vi "Periodic Tasks.vi"(8 "error in":errorcluster) -> ()   [LabVIEW 2015]
doc: "This VI runs in parallel to other tasks. It can contain as many user-defined periodic loops as you need. These can carry out PID or other sorts of timed response."
uses:
  <vilib>/Rock Robotics/WPI/Solenoid/Deprecated/WPI_SolenoidSetBool.vi
  <vilib>/Rock Robotics/WPI/Solenoid/Deprecated/WPI_SolenoidGetBool.vi
panel:
  in  "Left Art":dbl=0.5 format="%#_13g"
  in  "Right Art":dbl=0.5 format="%#_13g"
  in  "velocity_lower":dbl=1.0 format="%#_13g"
  in  "velocity_upper":dbl=1.0 format="%#_13g"
  out "error out":errorcluster
  # "change in time in milliseconds"
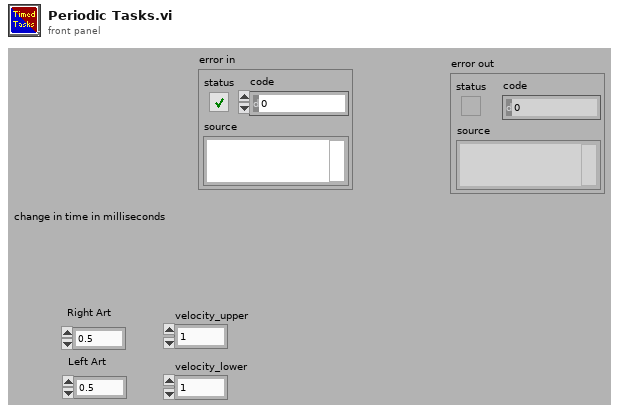
[diagram p1: front panel]
types:
  T1 = typedef "WPI_DigitalInputDevRef.ctl" = cluster{"DevStatus":errorcluster, "DIO Channel":T2}
  T2 = typedef "FPGA_DIOChannel.ctl" = enum8{"DIO 0", "DIO 1", "DIO 2", "DIO 3", "DIO 4", "DIO 5", "DIO 6", "DIO 7", "DIO 8", "DIO 9", "DIO MXP 0", "DIO MXP 1", "DIO MXP 2", "DIO MXP 3", "DIO MXP 4", "DIO MXP 5", "DIO MXP 6", "DIO MXP 7", "DIO MXP 8", "DIO MXP 9", "DIO MXP 10", "DIO MXP 11", "DIO MXP 12", "DIO MXP 13", "DIO MXP 14", "DIO MXP 15", "Invalid"}
  T3 = typedef "WPI_MotorControlDeviceRef.ctl" = cluster{"DeviceStatus":errorcluster, "Type":T4, "PWM":cluster{"PWM Channel":T5, "DeadBand":T6}, "CAN":cluster{"Device Number":u8, "Control Mode":T7, "Semaphore":T8, "Max Vout":dbl, "TalonSRX Control Mode":T9}, "Invert":bool}
  T4 = typedef "WPI_MotorControlType.ctl" = enum16{"PWM", "CAN", "CANTalonSRX"}
  T5 = typedef "FPGA_DIOPWMChannel.ctl" = enum8{"PWM 0", "PWM 1", "PWM 2", "PWM 3", "PWM 4", "PWM 5", "PWM 6", "PWM 7", "PWM 8", "PWM 9", "PWM MXP 0", "PWM MXP 1", "PWM MXP 2", "PWM MXP 3", "PWM MXP 4", "PWM MXP 5", "PWM MXP 6", "PWM MXP 7", "PWM MXP 8", "PWM MXP 9", "Invalid"}
  T6 = typedef "WPI_PWMDeadband.ctl" = cluster{"Name":string, "maxPositivePwm":i32, "minPositivePwm":i32, "centerPwm":i32, "maxNegativePwm":i32, "minNegativePwm":i32, "angularRange":u16}
  T7 = typedef "WPI_CANJaguar_ControlMode.ctl" = enum8{"Percent VBus", "Current", "Speed", "Position", "Voltage"}
  T8 = typedef "Semaphore RefNum" = refnum<k1>
  T9 = typedef "WPI_CANTalonSRX_APIControlMode.ctl" = enum8{"Percent VBus", "Speed", "Position", "Slave", "Unchanged / Invalid", "Voltage Compensation", "Current", "Motion Profile"}
  T10 = typedef "WPI_EncoderDevRef.ctl" = cluster{"DevStatus":errorcluster, "EncoderIndex":T11, "CounterIndex":T12, "DistancePerCount":dbl, "Decoding Type":T13}
  T11 = typedef "FPGA_EncoderIdx.ctl" = enum8{"Enc 0", "Enc 1", "Enc 2", "Enc 3", "Enc 4", "Enc 5", "Enc 6", "Enc 7", "Invalid"}
  T12 = typedef "FPGA_CounterCtrSystemIndex.ctl" = enum8{"Ctr 0", "Ctr 1", "Ctr 2", "Ctr 3", "Ctr 4", "Ctr 5", "Ctr 6", "Ctr 7", "Invalid"}
  T13 = typedef "WPI_EncoderType.ctl" = enum16{"1x", "2x", "4x"}
  T14 = typedef "WPI_DriverStationRobotMode2.ctl" = enum16{"Autonomous Disabled", "Autonomous Enabled", "Teleop Disabled", "Teleop Enabled", "Disconnected", "Finish", "Test Disabled", "Test Enabled", "Emergency Stopped"}
  T15 = typedef "WPI_SolenoidDevRef.ctl" = cluster{"DevStatus":errorcluster, "Pneumatics Control Module":u8, "Forward Solenoid Channel":T16, "Reverse Solenoid Channel":T16}
  T16 = typedef "WPI_SolenoidChannel.ctl" = enum8{"Solenoid 0", "Solenoid 1", "Solenoid 2", "Solenoid 3", "Solenoid 4", "Solenoid 5", "Solenoid 6", "Solenoid 7", "Invalid"}
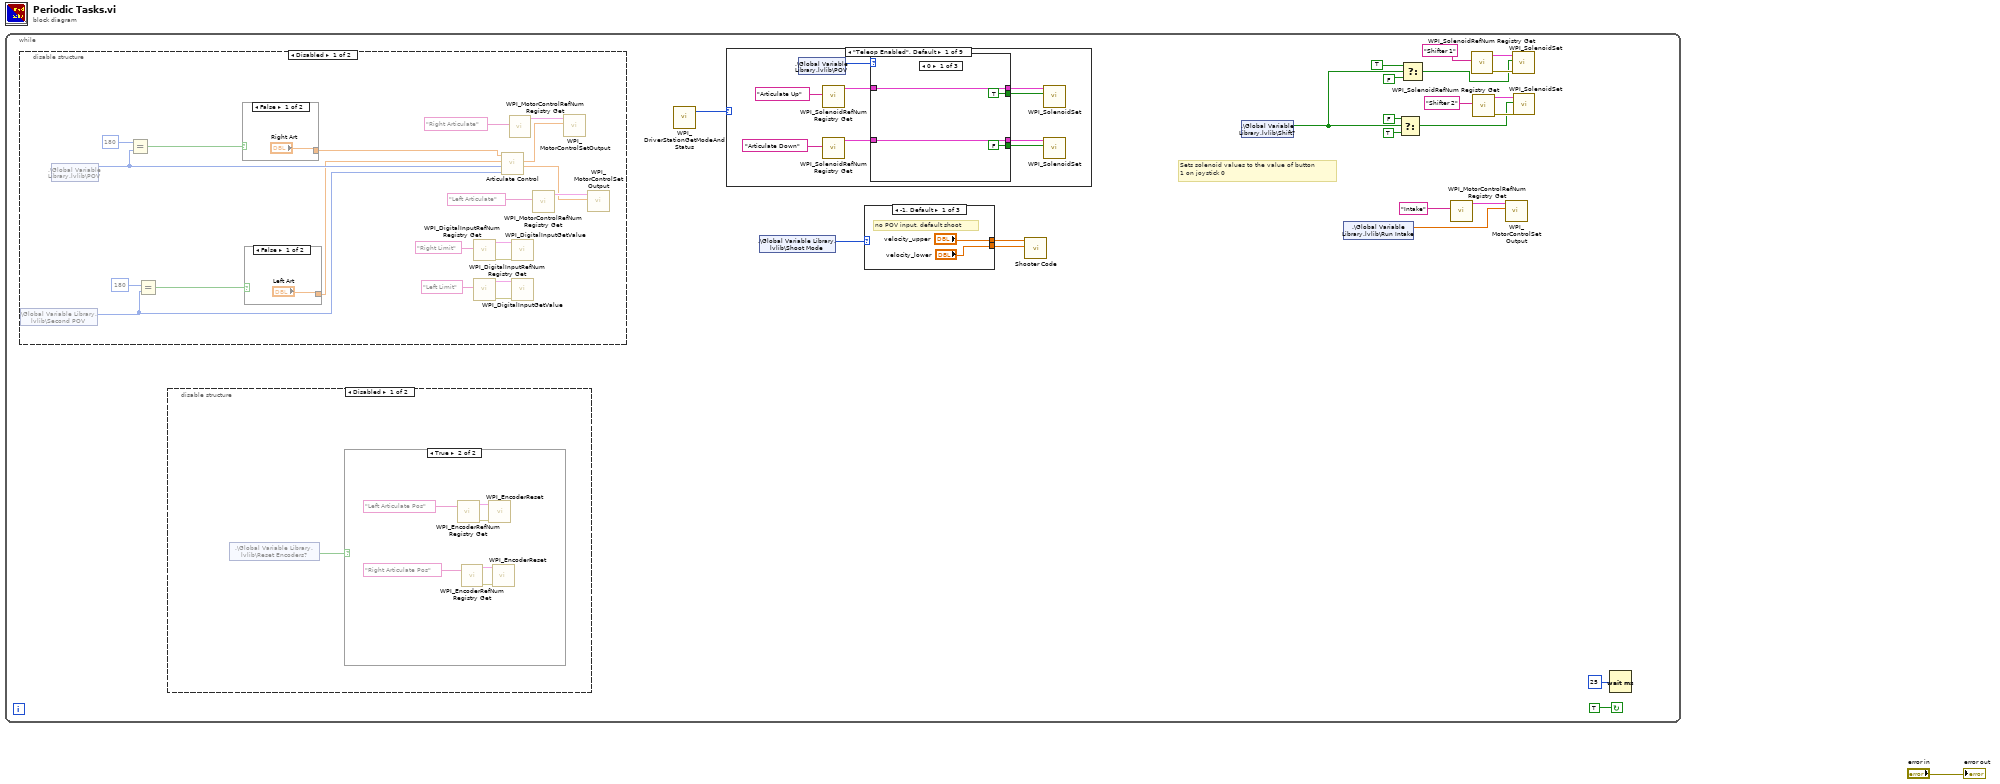
[diagram p0: block diagram]
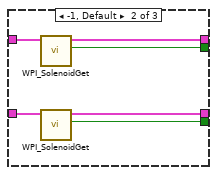
[diagram p2: hidden frame]
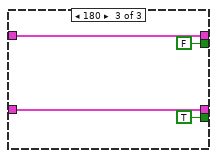
[diagram p3: hidden frame]
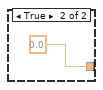
[diagram p14: hidden frame]
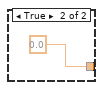
[diagram p15: hidden frame]
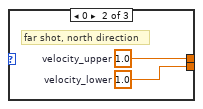
[diagram p17: hidden frame]
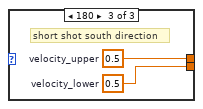
[diagram p18: hidden frame]
diagram:
  n1 = while {
    stop <- TRUE continue-if-true
    # "Sets solenoid values to the value of button\n1 on joystick 0"
    n2 = disable-structure shown="Disabled" {
      frame Disabled {
        n3 = shared-variable ".\\Global Variable Library.lvlib\\Second POV"() -> (w70:i16)  [unwired: 1 in, 1 out]
        n4 = shared-variable ".\\Global Variable Library.lvlib\\POV"() -> (w65:i16)  [unwired: 1 in, 1 out]
        n5 = Equal?(x=i16 180, y=w65) -> (x = y?=w64:bool)
        n6 = Equal?(x=i16 180, y=w70) -> (x = y?=w69:bool)
        n7 = case shown="False" w64 {
          tunnel: ["Right Art" 0.0] -> w66
          frame False {
          }
          frame True {
          }
        }
        n8 = case shown="False" w69 {
          tunnel: ["Left Art" 0.0] -> w60
          frame False {
          }
          frame True {
          }
        }
        n9 = call <vilib>:"WPI_DigitalInputRefNum Registry Get.vi"("refnum name"="Right Limit") -> ("error out"=w54:errorcluster, "DigitalInputDevRef"=w55:T1)  [unwired: 9 in]
        n10 = call <vilib>:"WPI_DigitalInputRefNum Registry Get.vi"("refnum name"="Left Limit") -> ("error out"=w59:errorcluster, "DigitalInputDevRef"=w58:T1)  [unwired: 9 in]
        n11 = call "Articulate Control.vi"("Second POV"=w70, "POV"=w65, "Left Articulate Target"=w60, "Right Articulate Target"=w66) -> ("Left Art Output"=w61:dbl, "Right Art Output"=w68:dbl)  [unwired: 6 in]
        n12 = call <vilib>:"WPI_MotorControlRefNum Registry Get.vi"("refnum name"="Right Articulate") -> ("MotorControlDevRef"=w63:T3)  [unwired: 9 in, 1 out]
        n13 = call <vilib>:"WPI_DigitalInputGetValue.vi"("error in (no error)"=w54, "DigitalInputDevRef"=w55) -> ()  [unwired: 7 in, 3 out]
        n14 = call <vilib>:"WPI_DigitalInputGetValue.vi"("error in (no error)"=w59, "DigitalInputDevRef"=w58) -> ()  [unwired: 7 in, 3 out]
        n15 = call <vilib>:"WPI_MotorControlRefNum Registry Get.vi"("refnum name"="Left Articulate") -> ("MotorControlDevRef"=w72:T3)  [unwired: 9 in, 1 out]
        n16 = call <vilib>:"WPI_MotorControlSetOutput.vi"("Output"=w68, "MotorControlDevRef"=w63) -> ()  [unwired: 7 in, 3 out]
        n17 = call <vilib>:"WPI_MotorControlSetOutput.vi"("Output"=w61, "MotorControlDevRef"=w72) -> ()  [unwired: 7 in, 3 out]
      }
      frame Enabled {
      }
    }
    n18 = disable-structure shown="Disabled" {
      frame Disabled {
        n19 = shared-variable ".\\Global Variable Library.lvlib\\Reset Encoders?"() -> (w47:bool)  [unwired: 1 in, 1 out]
        n20 = case shown="True" w47 {
          frame False {
          }
          frame True {
            n21 = call <vilib>:"WPI_EncoderRefNum Registry Get.vi"("refnum name"="Left Articulate Pos") -> ("error out"=w53:errorcluster, "EncoderDevRef"=w52:T10)  [unwired: 9 in]
            n22 = call <vilib>:"WPI_EncoderRefNum Registry Get.vi"("refnum name"="Right Articulate Pos") -> ("error out"=w48:errorcluster, "EncoderDevRef"=w49:T10)  [unwired: 9 in]
            n23 = call <vilib>:"WPI_EncoderReset.vi"("error in (no error)"=w53, "EncoderDevRef"=w52) -> ()  [unwired: 8 in, 2 out]
            n24 = call <vilib>:"WPI_EncoderReset.vi"("error in (no error)"=w48, "EncoderDevRef"=w49) -> ()  [unwired: 8 in, 2 out]
          }
        }
      }
      frame Enabled {
      }
    }
    n25 = call <vilib>:"WPI_DriverStationGetModeAndStatus.vi"() -> ("Robot Mode"=w2:T14)  [unwired: 10 in, 1 out]
    n26 = case shown="\"Teleop Enabled\", Default" w2 {
      frame "Teleop Enabled", Default {
        n27 = shared-variable ".\\Global Variable Library.lvlib\\POV"() -> (w32:i16)  [unwired: 1 in, 1 out]
        n28 = call <vilib>:"WPI_SolenoidRefNum Registry Get.vi"("refnum name"="Articulate Up") -> ("SolenoidDevRef"=w24:T15)  [unwired: 9 in, 1 out]
        n29 = call <vilib>:"WPI_SolenoidRefNum Registry Get.vi"("refnum name"="Articulate Down") -> ("SolenoidDevRef"=w31:T15)  [unwired: 9 in, 1 out]
        n30 = case shown="0" w32 {
          tunnel: w31 -> [w36 w42 w44]
          tunnel: [w36 w41 w44] -> w30
          tunnel: [FALSE ("Value") w40 TRUE ("Value")] -> w29
          tunnel: w24 -> [w35 w37 w45]
          tunnel: [w35 w38 w45] -> w25
          tunnel: [TRUE ("Value") w39 FALSE ("Value")] -> w26
          frame 0 {
          }
          frame -1, Default {
            n31 = call-poly <vilib>:"WPI_SolenoidGet.vi"("SolenoidDevRef"=w37) -> ("Value"=w39:bool, "SolenoidDevRef"=w38:T15)  [unwired: 8 in, 1 out]
            n32 = call-poly <vilib>:"WPI_SolenoidGet.vi"("SolenoidDevRef"=w42) -> ("Value"=w40:bool, "SolenoidDevRef"=w41:T15)  [unwired: 8 in, 1 out]
          }
          frame 180 {
          }
        }
        n33 = call-poly <vilib>:"WPI_SolenoidSet.vi"("Value"=w26, "SolenoidDevRef"=w25) -> ()  [unwired: 8 in, 2 out]
        n34 = call-poly <vilib>:"WPI_SolenoidSet.vi"("Value"=w29, "SolenoidDevRef"=w30) -> ()  [unwired: 8 in, 2 out]
      }
      frame "Disconnected" {
      }
      frame "Finish" {
      }
      frame "Test Disabled" {
      }
      frame "Test Enabled" {
      }
      frame "Emergency Stopped" {
      }
      frame "Teleop Disabled" {
      }
      frame "Autonomous Enabled" {
      }
      frame "Autonomous Disabled" {
      }
    }
    n35 = shared-variable ".\\Global Variable Library.lvlib\\Shoot Mode"() -> (w4:i16)  [unwired: 1 in, 1 out]
    n36 = case shown="-1, Default" w4 {
      tunnel: ["velocity_upper" w81 w83] -> w6
      tunnel: ["velocity_lower" w80 w82] -> w5
      frame -1, Default {
        # "no POV input, default shoot"
      }
      frame 0 {
        w80 = 1.0  # velocity_lower
        w81 = 1.0  # velocity_upper
        # "far shot, north direction"
      }
      frame 180 {
        w82 = 0.5  # velocity_lower
        w83 = 0.5  # velocity_upper
        # "short shot south direction"
      }
    }
    n37 = call "Shooter Code.vi"("velocity_lower"=w5, "velocity_upper"=w6) -> ()  [unwired: 10 in]
    n38 = shared-variable ".\\Global Variable Library.lvlib\\Shift?"() -> (w9:bool)  [unwired: 1 in, 1 out]
    n39 = shared-variable ".\\Global Variable Library.lvlib\\Run Intake"() -> (w3:dbl)  [unwired: 1 in, 1 out]
    n40 = Select(t=FALSE ("f"), s=w9, f=TRUE) -> (s? t:f=w10:bool)
    n41 = Select(t=TRUE, s=w9, f=FALSE) -> (s? t:f=w11:bool)
    n42 = call <vilib>:"WPI_MotorControlRefNum Registry Get.vi"("refnum name"="Intake") -> ("MotorControlDevRef"=w7:T3)  [unwired: 9 in, 1 out]
    n43 = call <vilib>:"WPI_SolenoidRefNum Registry Get.vi"("refnum name"="Shifter 1") -> ("error out"=w19:errorcluster, "SolenoidDevRef"=w18:T15)  [unwired: 9 in]
    n44 = call <vilib>:"WPI_SolenoidRefNum Registry Get.vi"("refnum name"="Shifter 2") -> ("error out"=w17:errorcluster, "SolenoidDevRef"=w16:T15)  [unwired: 9 in]
    n45 = call <vilib>:"WPI_MotorControlSetOutput.vi"("Output"=w3, "MotorControlDevRef"=w7) -> ()  [unwired: 7 in, 3 out]
    n46 = call-poly <vilib>:"WPI_SolenoidSet.vi"("error in (no error)"=w19, "Value"=w11, "SolenoidDevRef"=w18) -> ()  [unwired: 7 in, 2 out]
    n47 = call-poly <vilib>:"WPI_SolenoidSet.vi"("error in (no error)"=w17, "Value"=w10, "SolenoidDevRef"=w16) -> ()  [unwired: 7 in, 2 out]
    n48 = Wait (ms)(milliseconds to wait=u32 25) -> ()  [unwired: 1 out]
  }
  "error out" <- "error in"
